vi "Display Setup.vi"(0 "VISA resource name":refnum<visa-resource-name>, 1 "Enable Dots Only (F: Disable)":bool, 5 "Height (2: Large)":u16(ring)=2 items=["Small", "Medium", "Large"], 7 "Graticule Type (2: Full)":u16(ring)=2 items=["Crosshair", "Frame", "Full", "Grid"], 9 "Backlight (1: Medium)":u16(ring)=1 items=["Low", "Medium", "High"], 11 "error in (no error)":errorcluster, 12 "Graticule Visibility (50)":dbl=50.0, 13 "Waveform Visibility (70)":dbl=70.0) -> (4 "VISA resource name out":refnum<visa-resource-name>, 15 "error out":errorcluster)   [LabVIEW 2017, in "Scope.lvlib" / "Tektronix DPO MSO 2000 4000 Series.lvlib"]
doc: "Sets the display settings of the oscilloscope."
uses:
  Tektronix DPO MSO 2000 4000 Series.lvlib
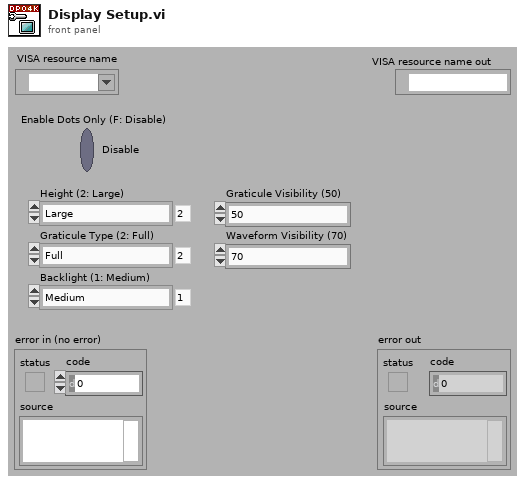
[diagram p1: front panel]
types:
  T1 = typedef "Scope.lvlib/Tektronix DPO MSO 2000 4000 Series.lvlib/Extended User Data.ctl" = cluster{"DPO MSO Series Model":u16}
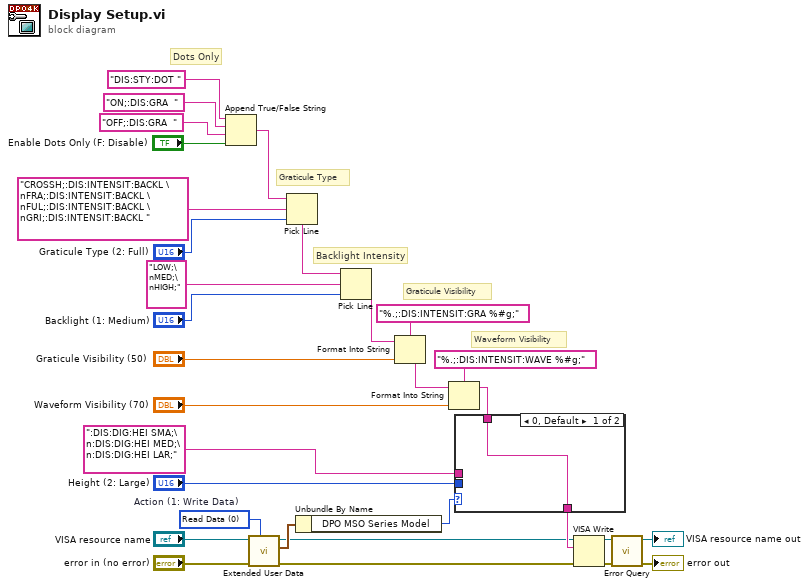
[diagram p0: block diagram]
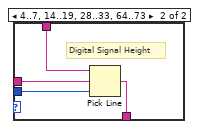
[diagram p2: hidden frame]
diagram:
  w6 = 0 items=["Read Data", "Write Data", "Clear Data", "Clear ALL Data"]  # Action (1: Write Data)
  # "Waveform Visibility"
  # "Graticule Visibility"
  # "Backlight Intensity"
  # "Graticule Type"
  # "Dots Only"
  n1 = Append True/False String(1:"Enable Dots Only (F: Disable)", 2:"OFF;:DIS:GRA  " ("false string"), 3:"ON;:DIS:GRA  " ("true string"), 4:"DIS:STY:DOT ") -> (0:w12:string)
  n2 = call "Extended User Data.vi"("Action (1: Write Data)"=w6, "error in (no error)"="error in (no error)", "VISA resource name"="VISA resource name") -> ("error out"=w2:errorcluster, "User Data Out"=w7:T1, "VISA resource name out"=w3:refnum<visa-resource-name>)  [unwired: 6 in]
  n3 = Pick Line(string ("")=w12, multi-line string="CROSSH;:DIS:INTENSIT:BACKL \nFRA;:DIS:INTENSIT:BACKL \nFUL;:DIS:INTENSIT:BACKL \nGRI;:DIS:INTENSIT:BACKL ", line index="Graticule Type (2: Full)") -> (output string=w25:string)
  n4 = Unbundle By Name(w7) -> ("DPO MSO Series Model"=w1:u16)
  n5 = Pick Line(string ("")=w25, multi-line string="LOW;\nMED;\nHIGH;", line index="Backlight (1: Medium)") -> (output string=w22:string)
  n6 = Format Into String(format string="%.;:DIS:INTENSIT:GRA %#g;", initial string=w22, "Graticule Visibility (50)") -> (resulting string=w19:string)  [unwired: 1 in, 1 out]
  n7 = Format Into String(format string="%.;:DIS:INTENSIT:WAVE %#g;", initial string=w19, "Waveform Visibility (70)") -> (resulting string=w9:string)  [unwired: 1 in, 1 out]
  n8 = case shown="0, Default" w1 {
    tunnel: "Height (2: Large)" -> [_ w36]
    tunnel: ":DIS:DIG:HEI SMA;\n:DIS:DIG:HEI MED;\n:DIS:DIG:HEI LAR;" ("multi-line string") -> [_ w35]
    tunnel: w9 -> [w32 w34]
    tunnel: [w32 w33] -> w8
    frame 0, Default {
    }
    frame 4..7, 14..19, 28..33, 64..73 {
      # "Digital Signal Height"
      n9 = Pick Line(string ("")=w34, multi-line string=w35, line index=w36) -> (output string=w33:string)
    }
  }
  n10 = VISA Write(VISA resource name=w3, write buffer=w8, error in (no error)=w2) -> (VISA resource name out=w16:refnum<visa-resource-name>, error out=w15:errorcluster)  [unwired: 1 out]
  n11 = call "Error Query.vi"("error in (no error)"=w15, "VISA resource name"=w16) -> ("error out"=→"error out":errorcluster, "VISA resource name out"=→"VISA resource name out":refnum<visa-resource-name>)  [unwired: 6 in, 2 out]
